vi "Self-Test.vi"(8 "error in (no error)":errorcluster, 9 "Device and Axis":string, 11 "VISA resource name":refnum<visa-resource-name>) -> (0 "error out":errorcluster, 1 "Self-Test Result Message":string, 3 "VISA resource name out":refnum<visa-resource-name>)   [LabVIEW 2015, in "Zaber A Series.lvlib"]
doc: "Sends an Echo command to the device with the text \"TEST OK\". This value should be read back in the data of the response. If not, there will be an error message.\n\nThis VI requires that the Initialize VI has been called with the same serial port."
uses:
  Zaber A Series.lvlib
  Private/All Commands.ctl
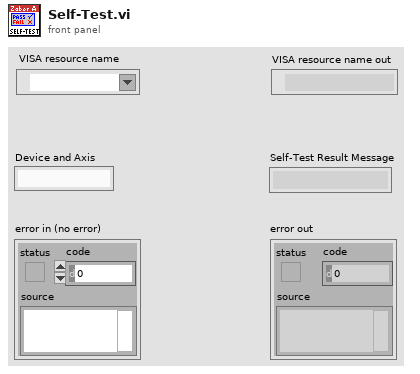
[diagram p1: front panel]
types:
  T1 = typedef "Zaber A Series.lvlib/All Commands.ctl" = string
  T2 = cluster{"Device":string, "Axis":string, "Reply Flag":string, "Status":string, "Warning Flags":string, "Data":string}
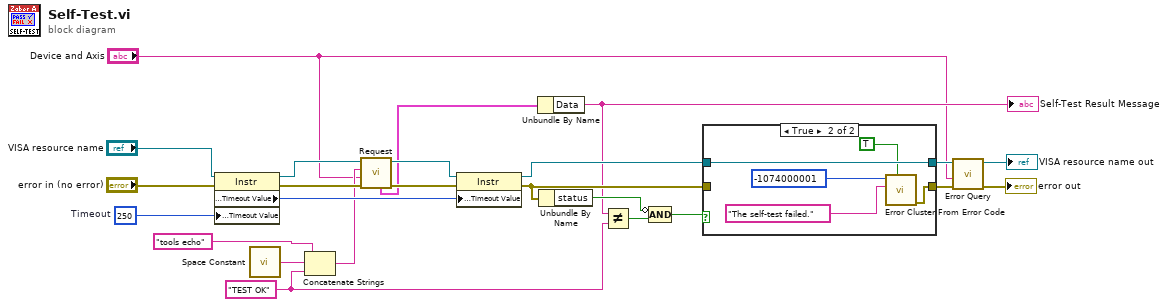
[diagram p0: block diagram]
diagram:
  w6 = "TEST OK" ("Data")
  w20 = u32 250  # Timeout
  n1 = property class="Instr"(reference="VISA resource name", error in="error in (no error)", "General Settings:Timeout Value"=w20) -> (reference out=w12:refnum<visa-resource-name>, error out=w10:errorcluster, "General Settings:Timeout Value"=w8:u32)
  n2 = call <vilib>:"Space Constant.vi"() -> ("String"=w4:string)
  n3 = Concatenate Strings(T1 "tools echo" ("Command List"), w4, w6) -> (w3:string)
  n4 = call "Request.vi"("error in (no error)"=w10, "Device and Axis"="Device and Axis", "Command String"=w3, "VISA resource name"=w12) -> ("error out"=w11:errorcluster, "VISA resource name out"=w7:refnum<visa-resource-name>, "First Response Bundle"=w1:T2)  [unwired: 2 in, 3 out]
  n5 = property class="Instr"(reference=w7, error in=w11, "General Settings:Timeout Value"=w8) -> (reference out=w19:refnum<visa-resource-name>, error out=w18:errorcluster)
  n6 = Unbundle By Name(w1) -> ("Data"=w9:string)
  "Self-Test Result Message" <- w9
  n7 = Unbundle By Name(w18) -> ("status"=w14:bool)
  n8 = Not Equal?(x=w9, y=w6) -> (x != y?=w15:bool)
  n9 = Compound Arithmetic op=AND(invert w14, w15) -> (w13:bool)
  n10 = case shown="True" w13 {
    tunnel: w19 -> [w26 w31]
    tunnel: w18 -> [w25 _]
    tunnel: [w25 w27] -> w17
    tunnel: [w26 w31] -> w16
    frame False {
    }
    frame True {
      n11 = call <vilib>:"Error Cluster From Error Code.vi"("show call chain? (False)"=TRUE, "error message (\"\")"="The self-test failed." ("Source (VI Name)"), "error code (0)"=-1074000001 ("Code")) -> ("error out"=w27:errorcluster)  [unwired: 6 in]
    }
  }
  n12 = call "Error Query.vi"("error in (no error)"=w17, "Device and Axis"="Device and Axis", "VISA resource name"=w16) -> ("error out"=→"error out":errorcluster, "VISA resource name out"=→"VISA resource name out":refnum<visa-resource-name>)  [unwired: 5 in, 2 out]
